vi "Continue Acquisition.vi"(8 "error in (no error)":errorcluster, 10 "Data Buffer":T1, 11 "Data Source in":refnum<class "Data Source.lvclass">) -> (0 "error out":errorcluster, 3 "Data Source out":refnum<class "Data Source.lvclass">)   [LabVIEW 2020, in "Data Source.lvlib" / "Data Source.lvclass"]
uses:
  Data Source.lvclass
  GPU FFT Calculator/GPU FFT Calculator/Data Source Buffer.ctl
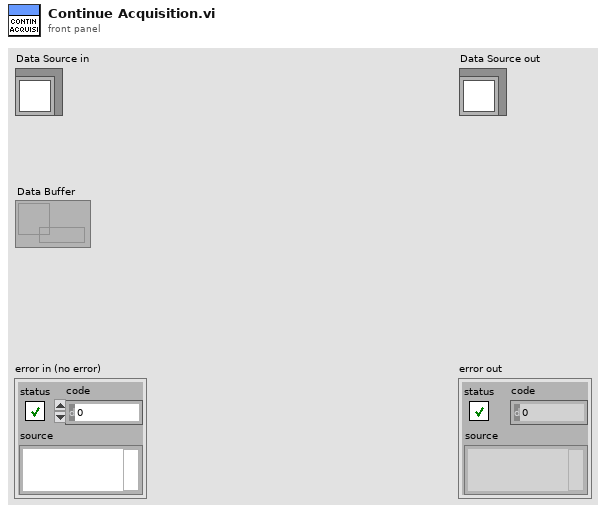
[diagram p1: front panel]
types:
  T1 = typedef "Data Source.lvlib/Data Source.lvclass/Data Source Buffer.ctl" = refnum<data-value>
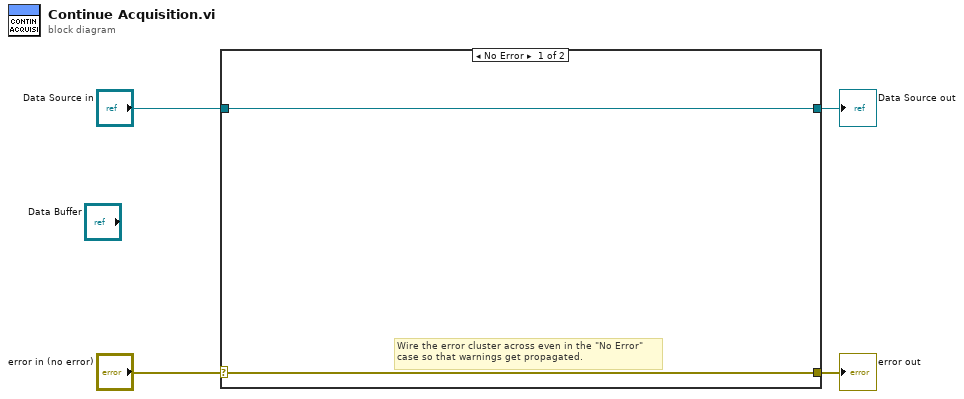
[diagram p0: block diagram]
diagram:
  n1 = case shown="No Error" "error in (no error)" {
    selector: "error in (no error)" -> [w5 w8]
    tunnel: [w5 w8] -> w3
    tunnel: [w6 w7] -> w1
    tunnel: "Data Source in" -> [w6 w7]
    frame No Error {
      # "Wire the error cluster across even in the \"No Error\"\ncase so that warnings get propagated."
    }
    frame Error {
    }
  }
  "error out" <- w3
  "Data Source out" <- w1
